vi "Disarm.vi"(8 "error in (no error)":errorcluster, 9 "Request type":T1=enum."User command", 11 "DAQmx Digitizer in":refnum<class "DAQmx Digitizer.lvclass">) -> (0 "error out":errorcluster, 2 "Armed":bool, 3 "DAQmx Digitizer out":refnum<class "DAQmx Digitizer.lvclass">)   [LabVIEW 2021, in "DAQmx Digitizer.lvclass"]
uses:
  DAQmx Digitizer.lvclass
  LabActor/Controllers/Process Controller/Request type.ctl
  Instruments/Pulse Driver/Lockin Digitizer Driver/Lockin Digitizer Driver.lvclass
  DAQmx Digitizer.lvclass/DAQmx Digitizer.ctl
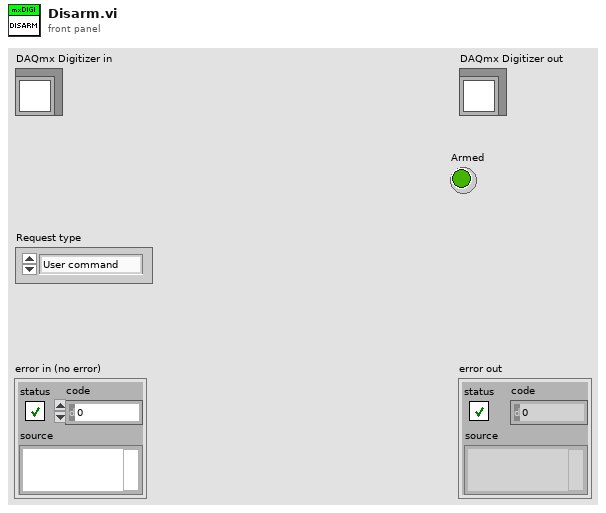
[diagram p1: front panel]
types:
  T1 = typedef "Request type.ctl" = enum16{"Process complete", "User command", "Auto-restart", "Error"}
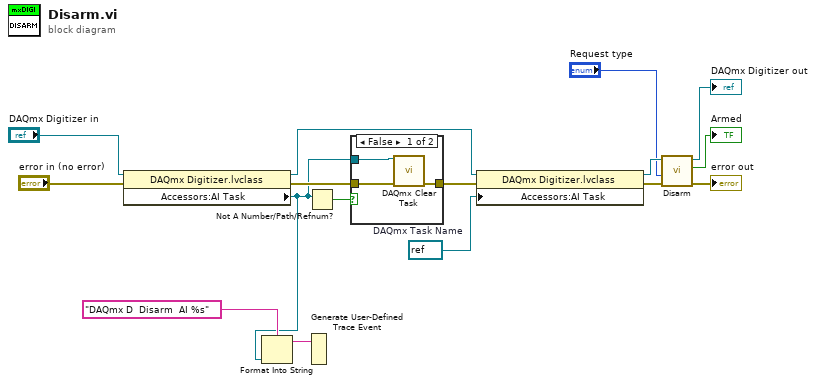
[diagram p0: block diagram]
diagram:
  w1 = refnum<k21> refnum  # DAQmx Task Name
  n1 = property class="DAQmx Digitizer.lvclass"(reference="DAQmx Digitizer in", error in="error in (no error)") -> (reference out=w8:refnum<class "DAQmx Digitizer.lvclass">, error out=w12:errorcluster, "Accessors:AI Task"=w3:refnum<k21>)
  n2 = Format Into String(format string="DAQmx D  Disarm  AI %s" ("string"), w3) -> (resulting string=w4:string)  [unwired: 2 in, 1 out]
  n3 = Generate User-Defined Trace Event(2:w4) -> ()  [unwired: 1 in]
  n4 = Not A Number/Path/Refnum?(number/path/refnum=w3) -> (NaN/Path/Refnum?=w13:bool)
  n5 = case shown="False" w13 {
    tunnel: w3 -> [w19 _]
    tunnel: w12 -> [w18 w20]
    tunnel: [w17 w20] -> w11
    frame False {
      n6 = call <vilib>:"DAQmx Clear Task.vi"("task in"=w19, "error in"=w18) -> ("error out"=w17:errorcluster)  [unwired: 13 out]
    }
    frame True {
    }
  }
  n7 = property class="DAQmx Digitizer.lvclass"(reference=w8, error in=w11, "Accessors:AI Task"=w1) -> (reference out=w7:refnum<class "DAQmx Digitizer.lvclass">, error out=w6:errorcluster)
  n8 = call-parent "Disarm.vi"("error in (no error)"=w6, "Request type"="Request type", "Pulse Driver in"=w7) -> ("error out"=→"error out":errorcluster, "Armed"=→"Armed":bool, "Pulse Driver out"=→"DAQmx Digitizer out":refnum<class "DAQmx Digitizer.lvclass">)  [unwired: 6 in]
